vi "Read Name.vi"(8 "error in (no error)":errorcluster, 11 "PluginInterface in":refnum<class "PluginInterface.lvclass">) -> (0 "error out":errorcluster, 2 "Name":string, 3 "PluginInterface out":refnum<class "PluginInterface.lvclass">)   [LabVIEW 2013, in "PluginInterface.lvlib" / "PluginInterface.lvclass"]
uses:
  PluginInterface.lvclass
  PluginInterface.lvclass/PluginInterface.ctl
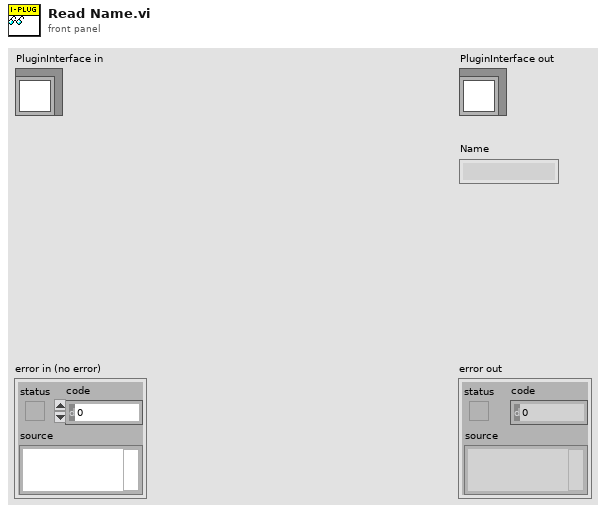
[diagram p1: front panel]
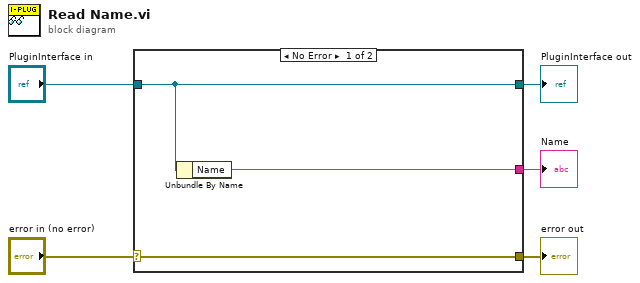
[diagram p0: block diagram]
diagram:
  n1 = case shown="No Error" "error in (no error)" {
    selector: "error in (no error)" -> [w8 w9]
    tunnel: [w8 w9] -> w4
    tunnel: [w7 w10] -> w2
    tunnel: "PluginInterface in" -> [w7 w10]
    tunnel: [w6 _] -> w1
    frame No Error {
      n2 = Unbundle By Name(w7) -> ("Name"=w6:string)
    }
    frame Error {
    }
  }
  "error out" <- w4
  "PluginInterface out" <- w2
  "Name" <- w1
